vi "ReadAttributeTest.vi"() -> ()   [LabVIEW 2013, in "examples.lvlib"]
uses:
  examples.lvlib
  vis/lv-2013/tango_vi.llb/ReadDoubleSpectrumAttribute.vi
  vis/lv-2013/tango_vi.llb/ReadDoubleImageAttribute.vi
  vis/lv-2013/tango_vi.llb/ReadLongSpectrumAttribute.vi
  vis/lv-2013/tango_vi.llb/ReadLongImageAttribute.vi
  vis/lv-2013/tango_vi.llb/ReadShortSpectrumAttribute.vi
  vis/lv-2013/tango_vi.llb/ReadShortImageAttribute.vi
  vis/lv-2013/tango_vi.llb/_TangoReadFloatScalarAttribute.vi
  vis/lv-2013/tango_vi.llb/_TangoReadLongScalarAttribute.vi
  vis/lv-2013/tango_vi.llb/_TangoReadShortScalarAttribute.vi
  vis/lv-2013/tango_vi.llb/_TangoReadLong64ScalarAttribute.vi
  vis/lv-2013/tango_vi.llb/_TangoReadBooleanScalarAttribute.vi
  vis/lv-2013/tango_vi.llb/_TangoReadStateScalarAttribute.vi
  vis/lv-2013/tango_vi.llb/_TangoReadStringScalarAttribute.vi
  vis/lv-2013/tango_vi.llb/_TangoReadDoubleScalarAttribute.vi
  vis/lv-2013/tango_vi.llb/_TangoReadULong64ScalarAttribute.vi
  vis/lv-2013/tango_vi.llb/_TangoReadULongScalarAttribute.vi
  vis/lv-2013/tango_vi.llb/_TangoReadUShortScalarAttribute.vi
  vis/lv-2013/tango_vi.llb/_TangoReadUCharScalarAttribute.vi
  vis/lv-2013/tango_vi.llb/tango.lvlib
panel:
  out "?":bool
  out "?":bool
  out "?":bool
  out "?":bool
  out "?":bool
  out "State Color":u32(colorbox)=16448250
  out "State Name":string
  out "?":bool
  out "?":string
  out "?":i32[](graph)
  out "?":string
  out "?":u64(graph)
  out "?":bool
  out "?":string
  out "?":i64(graph)
  out "?":bool
  out "?":string
  out "?":u32(graph)
  out "?":bool
  out "?":string
  out "?":u16(graph)
  out "?":bool
  out "?":string
  out "?":u8(graph)
  out "?":string
  out "scalar attr. value 5":dbl(graph)
  out "?":string
  out "scalar attr. value 4":sgl(graph)
  out "?":string
  out "?":bool
  out "?":string
  out "?":string
  out "scalar attr. value 3":i32(graph)
  out "spectrum attr. value 3":i16[](graph)
  out "?":bool
  out "?":string
  out "image attr. value":i16[][](graph)
  out "?":bool
  out "?":string
  out "image attr. value":i32[][](graph)
  out "?":bool
  out "?":string
  out "?":string
  out "scalar attr. value 2":i16(graph)
  out "?":bool
  out "?":string
  out "?":i16(graph)
  out "?":bool
  out "?":string
  out "?":bool
  out "?":string
  out "?":bool
  out "image attr. value":dbl[][](graph)
  out "?":dbl[](graph)
  out "?":string
  in  "<TangoTest> device name":string="sys/tg_test/1"
  # "TANGO  Binding for LabVIEW - ReadAttribute example"
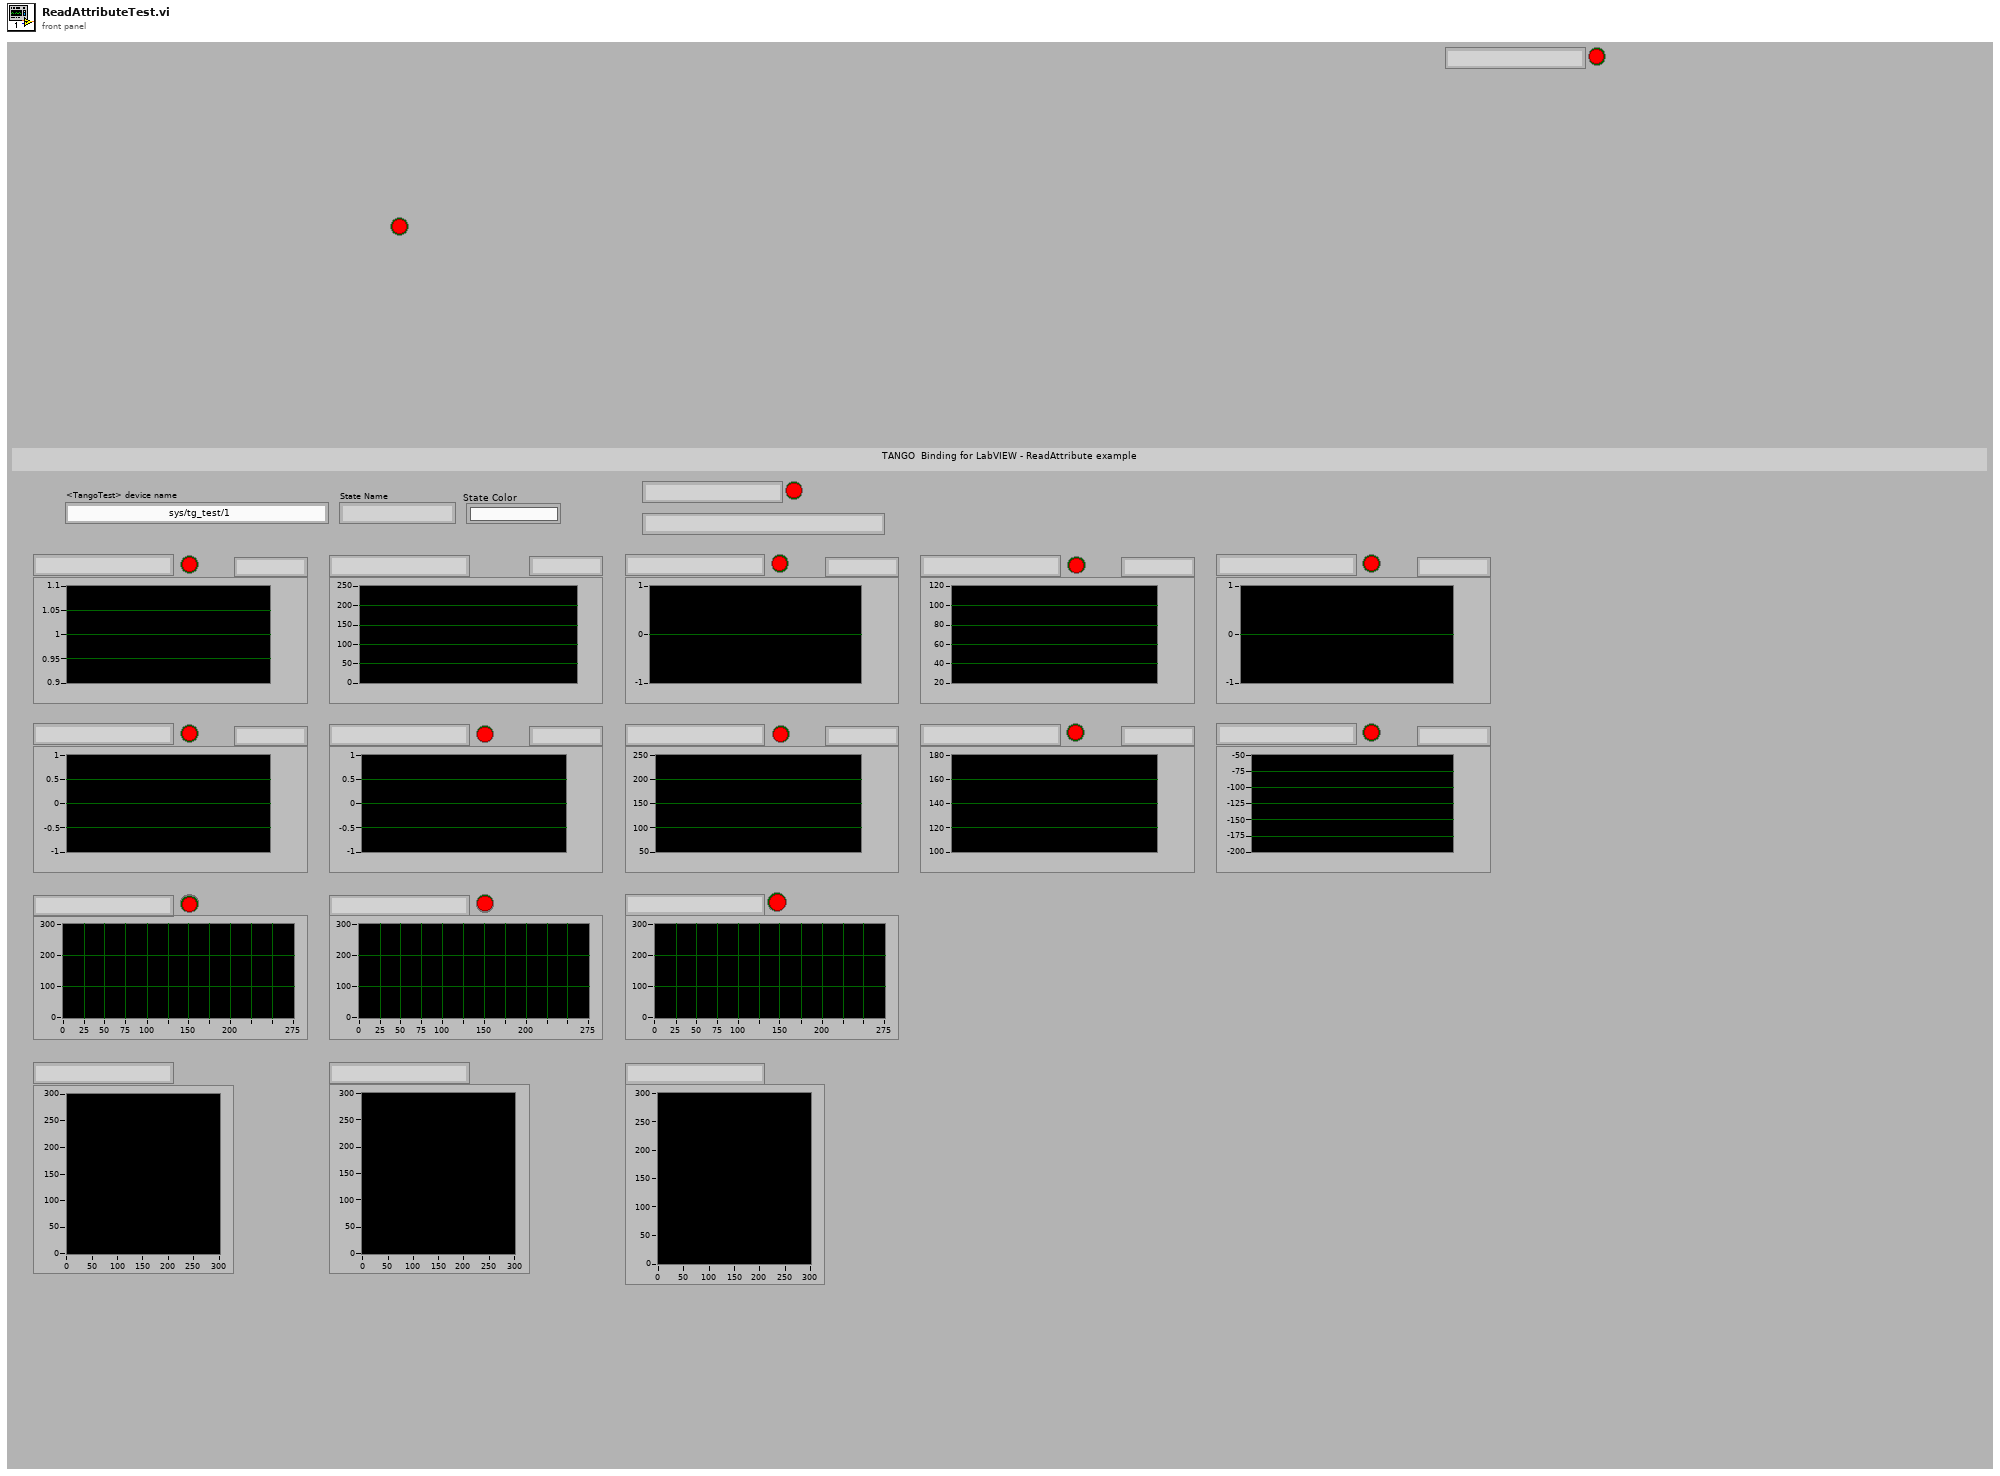
[diagram p1: front panel]
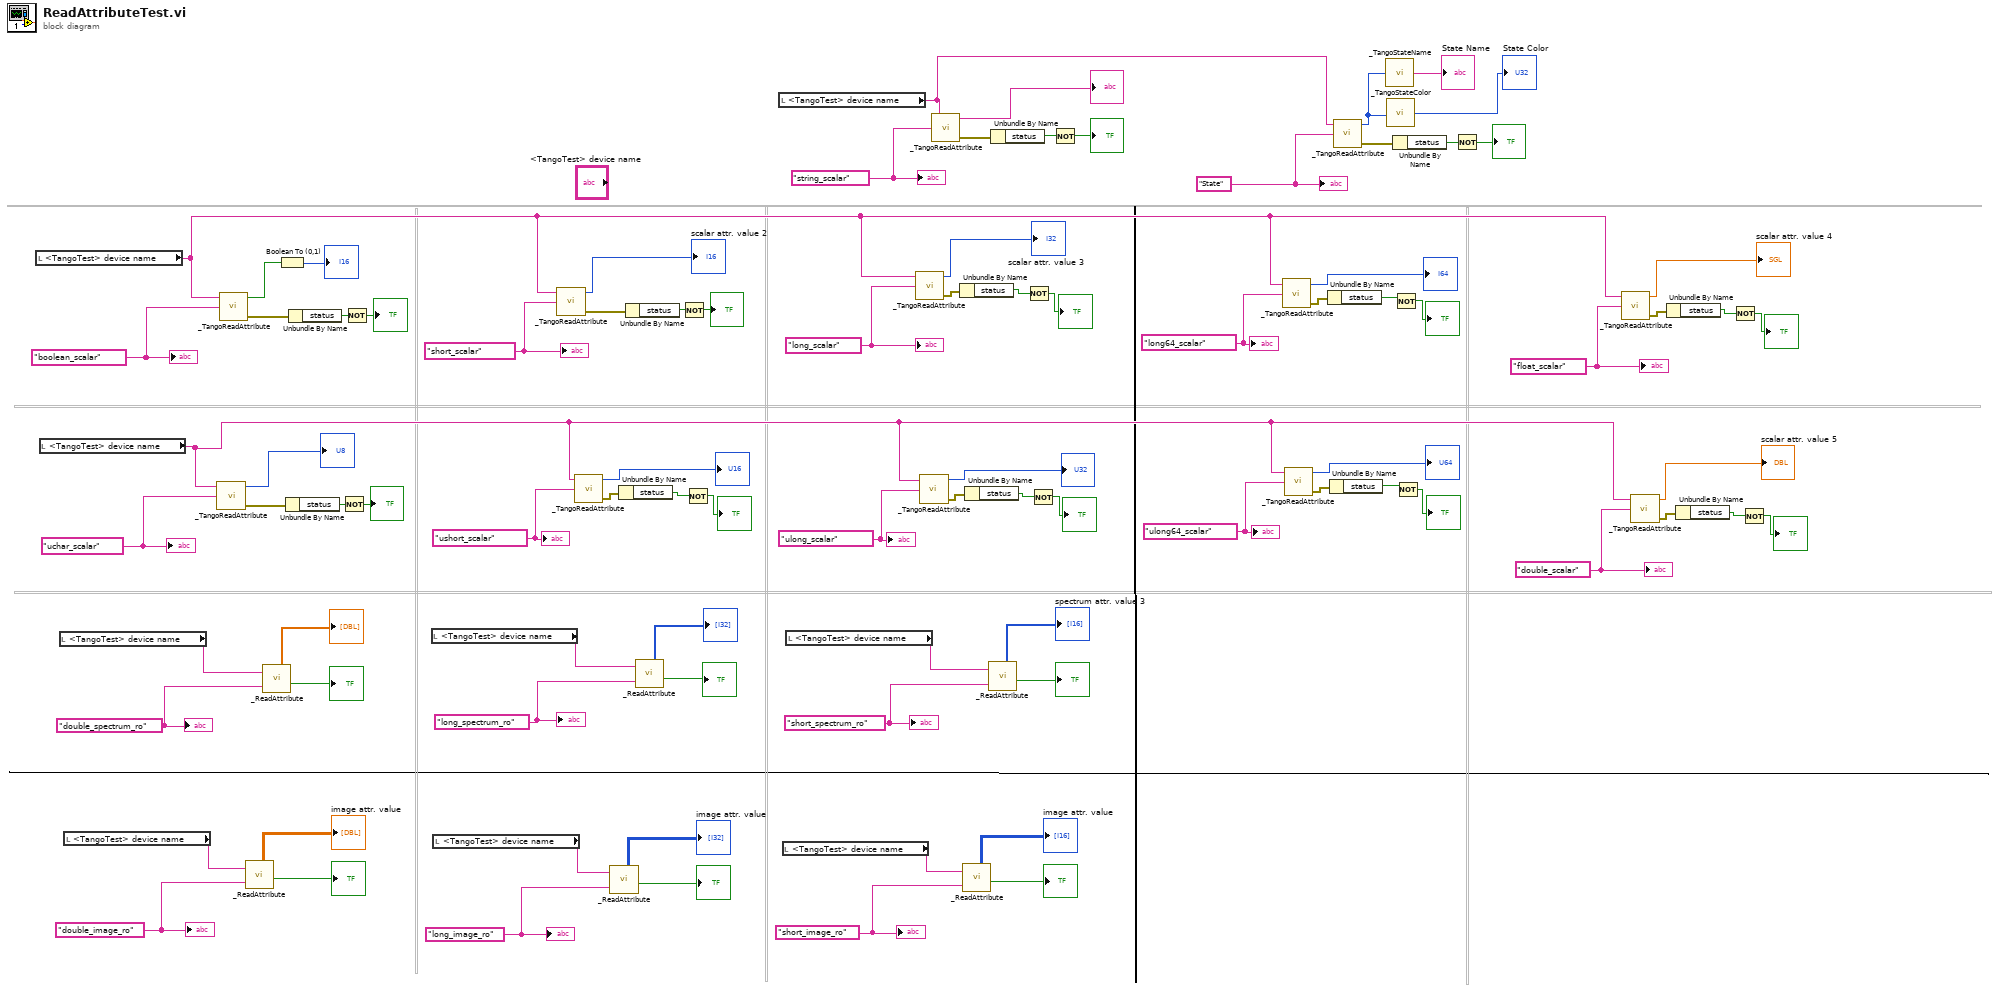
[diagram p0: block diagram]
diagram:
  w31 = "State"
  w34 = "ulong64_scalar"
  w39 = "long64_scalar"
  w44 = "ulong_scalar"
  w50 = "ushort_scalar"
  w53 = "uchar_scalar"
  w3 = "double_scalar"
  w11 = "float_scalar"
  w71 = "string_scalar"
  w2 = "long_scalar"
  w79 = "short_spectrum_ro"
  w81 = "short_image_ro" ("attr_name")
  w83 = "long_image_ro" ("attr_name")
  w20 = "short_scalar"
  w85 = "long_spectrum_ro"
  w87 = "double_image_ro" ("attr_name")
  w59 = "boolean_scalar"
  w90 = "double_spectrum_ro"
  n1 = local read "<TangoTest> device name"() -> (w10:string)
  n2 = local read "<TangoTest> device name"() -> (w4:string)
  n3 = local read "<TangoTest> device name"() -> (w77:string)
  n4 = local read "<TangoTest> device name"() -> (w76:string)
  n5 = call-poly "_TangoReadAttribute.vi"("attribute name"=w53, "device name"=w4) -> ("error out"=w56:errorcluster, "value"=→"?":u8)  [unwired: 1 in, 1 out]
  n6 = call-poly "_TangoReadAttribute.vi"("attribute name"=w59, "device name"=w10) -> ("error out"=w65:errorcluster, "value"=w58:bool)  [unwired: 1 in, 1 out]
  n7 = call-poly "_ReadAttribute.vi"("device name"=w76, "attribute name"=w87) -> ("value"=→"image attr. value":dbl[][], "success"=→"?":bool)  [unwired: 4 out]
  n8 = call-poly "_ReadAttribute.vi"("device name"=w77, "attribute name"=w90) -> ("value"=→"?":dbl[], "success"=→"?":bool)  [unwired: 4 out]
  n9 = Boolean To (0,1)(Boolean=w58) -> (0, 1=→"?":i16)
  n10 = Unbundle By Name(w56) -> ("status"=w54:bool)
  n11 = Unbundle By Name(w65) -> ("status"=w63:bool)
  n12 = Not(x=w54) -> (.not. x?=→"?":bool)
  n13 = Not(x=w63) -> (.not. x?=→"?":bool)
  n14 = local read "<TangoTest> device name"() -> (w75:string)
  n15 = local read "<TangoTest> device name"() -> (w74:string)
  n16 = call-poly "_TangoReadAttribute.vi"("attribute name"=w20, "device name"=w10) -> ("error out"=w23:errorcluster, "value"=→"scalar attr. value 2":i16)  [unwired: 1 in, 1 out]
  n17 = call-poly "_TangoReadAttribute.vi"("attribute name"=w50, "device name"=w4) -> ("error out"=w52:errorcluster, "value"=→"?":u16)  [unwired: 1 in, 1 out]
  n18 = call-poly "_ReadAttribute.vi"("device name"=w74, "attribute name"=w83) -> ("value"=→"image attr. value":i32[][], "success"=→"?":bool)  [unwired: 4 out]
  n19 = Unbundle By Name(w52) -> ("status"=w51:bool)
  n20 = Unbundle By Name(w23) -> ("status"=w21:bool)
  n21 = call-poly "_ReadAttribute.vi"("device name"=w75, "attribute name"=w85) -> ("value"=→"?":i32[], "success"=→"?":bool)  [unwired: 4 out]
  n22 = Not(x=w21) -> (.not. x?=→"?":bool)
  n23 = Not(x=w51) -> (.not. x?=→"?":bool)
  n24 = local read "<TangoTest> device name"() -> (w27:string)
  n25 = local read "<TangoTest> device name"() -> (w73:string)
  n26 = local read "<TangoTest> device name"() -> (w72:string)
  n27 = call-poly "_TangoReadAttribute.vi"("attribute name"=w2, "device name"=w10) -> ("error out"=w18:errorcluster, "value"=→"scalar attr. value 3":i32)  [unwired: 1 in, 1 out]
  n28 = call-poly "_TangoReadAttribute.vi"("attribute name"=w44, "device name"=w4) -> ("error out"=w46:errorcluster, "value"=→"?":u32)  [unwired: 1 in, 1 out]
  n29 = call-poly "_TangoReadAttribute.vi"("attribute name"=w71, "device name"=w27) -> ("error out"=w61:errorcluster, "value"=→"?":string)  [unwired: 1 in, 1 out]
  n30 = Unbundle By Name(w18) -> ("status"=w17:bool)
  n31 = call-poly "_ReadAttribute.vi"("device name"=w73, "attribute name"=w81) -> ("value"=→"image attr. value":i16[][], "success"=→"?":bool)  [unwired: 4 out]
  n32 = Unbundle By Name(w46) -> ("status"=w45:bool)
  n33 = call-poly "_ReadAttribute.vi"("device name"=w72, "attribute name"=w79) -> ("value"=→"spectrum attr. value 3":i16[], "success"=→"?":bool)  [unwired: 4 out]
  n34 = Unbundle By Name(w61) -> ("status"=w62:bool)
  n35 = Not(x=w17) -> (.not. x?=→"?":bool)
  n36 = Not(x=w45) -> (.not. x?=→"?":bool)
  n37 = Not(x=w62) -> (.not. x?=→"?":bool)
  n38 = call-poly "_TangoReadAttribute.vi"("attribute name"=w39, "device name"=w10) -> ("error out"=w41:errorcluster, "value"=→"?":i64)  [unwired: 1 in, 1 out]
  n39 = call-poly "_TangoReadAttribute.vi"("attribute name"=w34, "device name"=w4) -> ("error out"=w36:errorcluster, "value"=→"?":u64)  [unwired: 1 in, 1 out]
  n40 = Unbundle By Name(w41) -> ("status"=w40:bool)
  n41 = Unbundle By Name(w36) -> ("status"=w35:bool)
  n42 = call-poly "_TangoReadAttribute.vi"("attribute name"=w31, "device name"=w27) -> ("error out"=w29:errorcluster, "value"=w24:u32)  [unwired: 1 in, 1 out]
  n43 = call "_TangoStateName.vi"("State"=w24) -> ("State Name"=→"State Name":string)
  n44 = call "_TangoStateColor.vi"("State"=w24) -> ("State Color"=→"State Color":u32)
  n45 = Not(x=w40) -> (.not. x?=→"?":bool)
  n46 = Unbundle By Name(w29) -> ("status"=w30:bool)
  n47 = Not(x=w35) -> (.not. x?=→"?":bool)
  n48 = Not(x=w30) -> (.not. x?=→"?":bool)
  n49 = call-poly "_TangoReadAttribute.vi"("attribute name"=w11, "device name"=w10) -> ("error out"=w14:errorcluster, "value"=→"scalar attr. value 4":sgl)  [unwired: 1 in, 1 out]
  n50 = call-poly "_TangoReadAttribute.vi"("attribute name"=w3, "device name"=w4) -> ("error out"=w8:errorcluster, "value"=→"scalar attr. value 5":dbl)  [unwired: 1 in, 1 out]
  n51 = Unbundle By Name(w14) -> ("status"=w13:bool)
  n52 = Unbundle By Name(w8) -> ("status"=w7:bool)
  n53 = Not(x=w13) -> (.not. x?=→"?":bool)
  n54 = Not(x=w7) -> (.not. x?=→"?":bool)
  "?" <- w90
  "?" <- w59
  "?" <- w87
  "?" <- w85
  "?" <- w20
  "?" <- w83
  "?" <- w81
  "?" <- w79
  "?" <- w2
  "?" <- w71
  "?" <- w11
  "?" <- w3
  "?" <- w53
  "?" <- w50
  "?" <- w44
  "?" <- w39
  "?" <- w34
  "?" <- w31
